vi "Infrared Sensor value.vi"() -> ()   [LabVIEW 2011]
panel:
  in  "Infrared Sensor Value":dbl
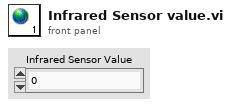
[diagram p1: front panel]
diagram:
